vi "Video Processing.vi"() -> ()   [LabVIEW 2014]
uses:
  Global.vi
  <vilib>/vision/NI_Vision_Development_Module.lvlib
panel:
  out "Video Loop":errorcluster
  out "Motion Flow":T1(plugin-control)
  out "Number of Particles before":i32
  out "Processed Image":T1(plugin-control)
  out "Number of Particles after":i32
  in  "Number of Erosion":i32=30
  out "x-y":u32=48
  out "Read Video":errorcluster
  in  "milliseconds to wait":u32
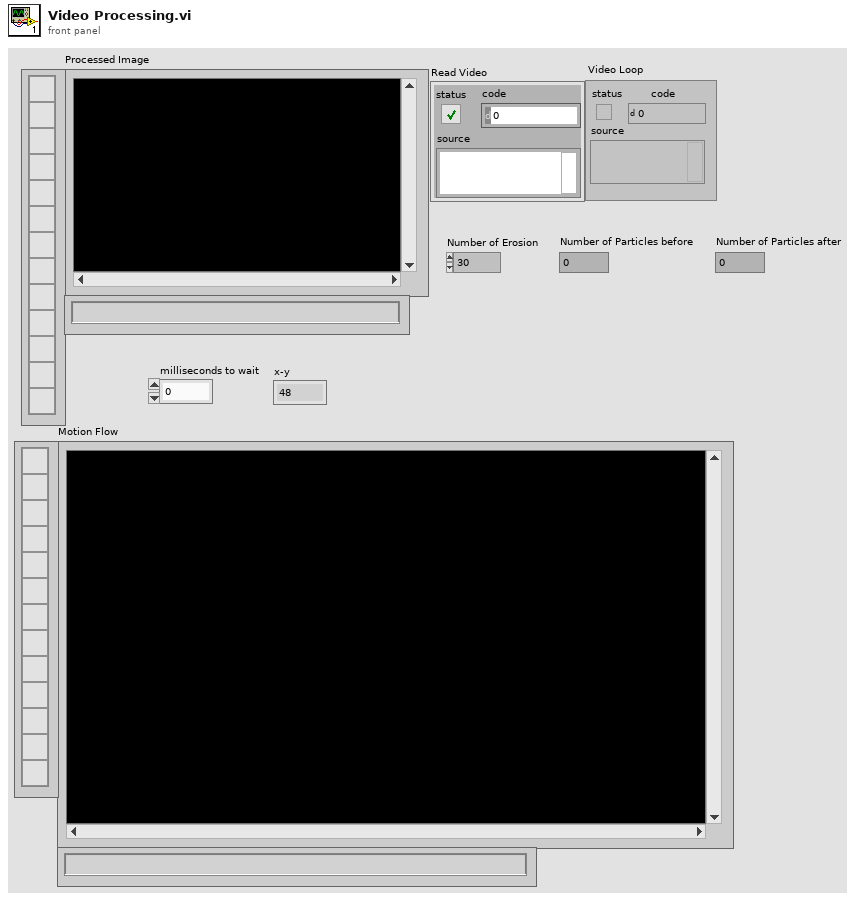
[diagram p1: front panel]
types:
  T1 = typedef "IMAQ Image.ctl" = refnum<image>
  T2 = typedef "Image Type" = u32
  T3 = cluster{"Numeric":dbl, "Numeric":dbl, "Numeric":dbl, "Numeric":dbl}
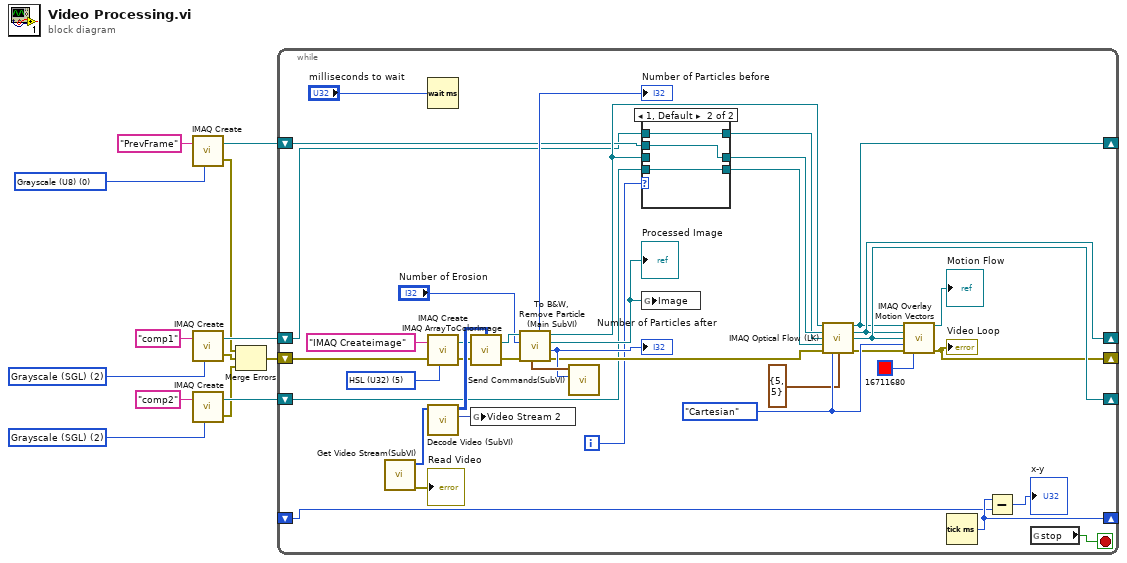
[diagram p0: block diagram]
diagram:
  w7 = T2 2 items=["Grayscale (U8)", "Grayscale (I16)", "Grayscale (SGL)", "Complex (CSG)", "RGB (U32)", "HSL (U32)", "RGB (U64)", "Grayscale (U16)"] ("Image Type")
  w12 = T2 2 items=["Grayscale (U8)", "Grayscale (I16)", "Grayscale (SGL)", "Complex (CSG)", "RGB (U32)", "HSL (U32)", "RGB (U64)", "Grayscale (U16)"] ("Image Type")
  w13 = T2 0 items=["Grayscale (U8)", "Grayscale (I16)", "Grayscale (SGL)", "Complex (CSG)", "RGB (U32)", "HSL (U32)", "RGB (U64)", "Grayscale (U16)"] ("Image Type")
  n1 = call "IMAQ Create"("Image Name"="PrevFrame", "Image Type"=w13) -> ("New Image"=w11:T1, "error out"=w2:errorcluster)  [unwired: 3 in]
  n2 = call "IMAQ Create"("Image Name"="comp1", "Image Type"=w7) -> ("New Image"=w5:T1, "error out"=w3:errorcluster)  [unwired: 3 in]
  n3 = call "IMAQ Create"("Image Name"="comp2", "Image Type"=w12) -> ("New Image"=w8:T1, "error out"=w4:errorcluster)  [unwired: 3 in]
  n4 = Merge Errors(w2, w3, w4) -> (w1:errorcluster)
  n5 = while {
    shift-right: [w44] -> _
    shift-left: _ -> [w43]
    shift-right: [w25] -> _
    shift-left: w1 -> [w33]
    shift-right: [w23] -> _
    shift-left: w11 -> [w19]
    shift-right: [w29] -> _
    shift-left: w5 -> [w14]
    shift-right: [w30] -> _
    shift-left: w8 -> [w18]
    i -> [w22]
    stop <- w34 stop-if-true
    w31 = enum16{"Cartesian", "Polar"}."Cartesian" ("Velocity Representation")
    w50 = T2 5 items=["Grayscale (U8)", "Grayscale (I16)", "Grayscale (SGL)", "Complex (CSG)", "RGB (U32)", "HSL (U32)", "RGB (U64)", "Grayscale (U16)"] ("Image Type")
    n6 = call "Get Video Stream(SubVI).vi"() -> ("error out"=→"Read Video":errorcluster, "ImgData"=w51:u8[])  [unwired: 10 in]
    n7 = Wait (ms)(milliseconds to wait="milliseconds to wait") -> ()  [unwired: 1 out]
    n8 = call "IMAQ Create"("Image Name"="IMAQ Createimage", "Image Type"=w50, "error in (no error)"=w33) -> ("New Image"=w46:T1, "error out"=w45:errorcluster)  [unwired: 2 in]
    n9 = call "Decode Video (SubVI).vi"("ImgData"=w51) -> ("new picture"=w41:picture, "Array"=w47:u32[][])  [unwired: 9 in]
    n10 = call "IMAQ ArrayToColorImage"("Image Pixels (U32)"=w47, "Image"=w46, "error in (no error)"=w45) -> ("Image Out"=w40:T1, "error out"=w39:errorcluster)  [unwired: 2 in]
    n11 = global write "Global.vi" "Video Stream 2"(w41) -> ()
    n12 = call "To B&W, Remove Particle (Main SubVI).vi"("error in (no error)"=w39, "Number of Erosion"="Number of Erosion", "Refnum in"=w40) -> ("error out"=w32:errorcluster, "Number of Particles after"=w35:i32, "Image Out"=w27:T1, "Current Grayscale"=w20:T1, "Number of Particles before"=→"Number of Particles before":i32, "Cluster"=w37:T3)  [unwired: 2 in, 1 out]
    "Number of Particles after" <- w35
    "Processed Image" <- w27
    n13 = call "Send Commands(SubVI).vi"("Number of Particles after"=w35, "Cluster"=w37) -> ()  [unwired: 10 in]
    n14 = case shown="1, Default" w22 {
      tunnel: [w54 w58] -> w21
      tunnel: w20 -> [w54 _]
      tunnel: w19 -> [_ w58]
      tunnel: [w55 w57] -> w16
      tunnel: [w53 w56] -> w17
      tunnel: w14 -> [w55 w57]
      tunnel: w18 -> [w53 w56]
      frame 0 {
      }
      frame 1, Default {
      }
    }
    n15 = global write "Global.vi" "Image"(w27) -> ()
    n16 = call "IMAQ Optical Flow (LK)"("Current Frame"=w20, "Previous Frame"=w21, "Velocity Component 1 In"=w16, "Velocity Component 2 In"=w17, "error in (no error)"=w32, "Velocity Representation"=w31, "Window Size (15x15)"=cluster{"SizeX":i32, "SizeY":i32} {"SizeX"=5, "SizeY"=5}) -> ("Current Frame Out (dup)"=w23:T1, "Velocity Component 1 Out"=w29:T1, "Velocity Component 2 Out"=w30:T1, "error out"=w24:errorcluster)  [unwired: 5 in]
    n17 = call "IMAQ Overlay Motion Vectors"("Image"=w23, "Velocity Component 1"=w29, "Velocity Component 2"=w30, "Velocity Representation"=w31, "error in (no error)"=w24, "Color"=u32 16711680) -> ("Image Out"=→"Motion Flow":T1, "error out"=w25:errorcluster)  [unwired: 8 in]
    "Video Loop" <- w25
    n18 = Tick Count (ms)() -> (millisecond timer value=w44:u32)
    n19 = Subtract(x=w44, y=w43) -> (x-y=→"x-y":u32)
    n20 = global read "Global.vi" "stop"() -> (w34:bool)
  }
